vi "libssh2_channel_flush_stderr.vi"(8 "error in (no error)":errorcluster, 11 "channel":T1) -> (0 "error out":errorcluster)   [LabVIEW 2017, in "libssh2.lvlib"]
doc: "Flush the standard error buffer for a channel."
uses:
  libssh2.lvlib
  Channel Refnum.ctl
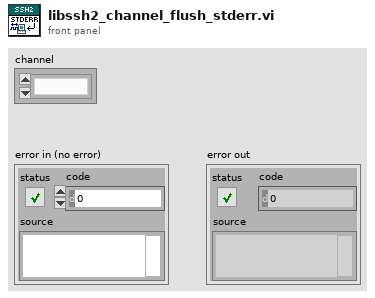
[diagram p1: front panel]
types:
  T1 = typedef "libssh2.lvlib/Channel Refnum.ctl" = refnum<k1>
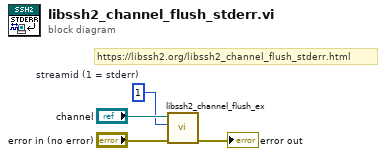
[diagram p0: block diagram]
diagram:
  w2 = 1  # streamid (1 = stderr)
  # "https://libssh2.org/libssh2_channel_flush_stderr.html"
  n1 = call "libssh2_channel_flush_ex.vi"("error in (no error)"="error in (no error)", "streamid"=w2, "channel"="channel") -> ("error out"=→"error out":errorcluster)  [unwired: 8 in]
